vi "Main_007.vi"() -> ()   [LabVIEW 2025]
uses:
  Utility/Universal Utility/TypeDefs_Utility/Cluster_Row-Column.ctl
  9e3f57c0-2ef8-4495-8287-c6a42a5fb955.vi
  Utility/Universal Utility/TypeDefs_Utility/ENUM_4 Directions U-D-L-R.ctl
  Utility/Universal Utility/TypeDefs_Utility/ENUM_8 Directions U-D-L-R.ctl
  <vilib>/gmath/NI_AAL_MathFunc.lvlib
panel:
  out "MATCH":bool
  in  "Select Data":enum32{"Example", "Puzzle"}(tab)
  in  "EX Target":u64=13
  in  "Example Input":u64=6
  in  "Puzzle Input":u64=10001
  in  "Puzzle Target":u64=104743
  out "Answer":u64
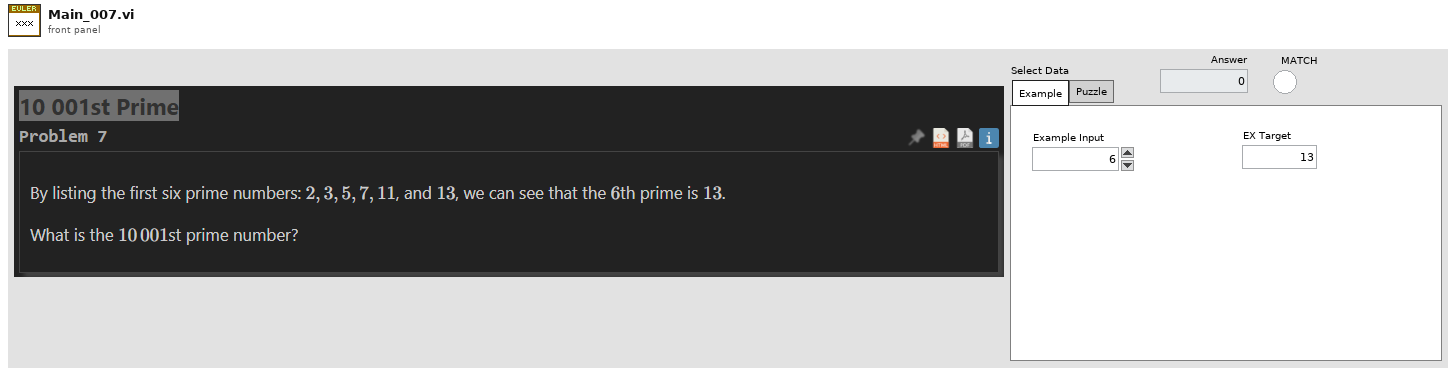
[diagram p1: front panel]
types:
  T1 = typedef "ENUM_8 Directions U-D-L-R.ctl" = enum16{"Up;-1,0", "Up-Right;-1,1", "Right;0,1", "Down-Right;1,1", "Down;1,0", "Down-Left;1,-1", "Left;0,-1", "Up-Left;-1,-1"}
  T2 = typedef "ENUM_4 Directions U-D-L-R.ctl" = enum16{"Up;-1,0", "Right;0,1", "Down;1,0", "Left;0,-1"}
  T3 = typedef "Cluster_Row-Column.ctl" = cluster{"R":i32, "C":i32}
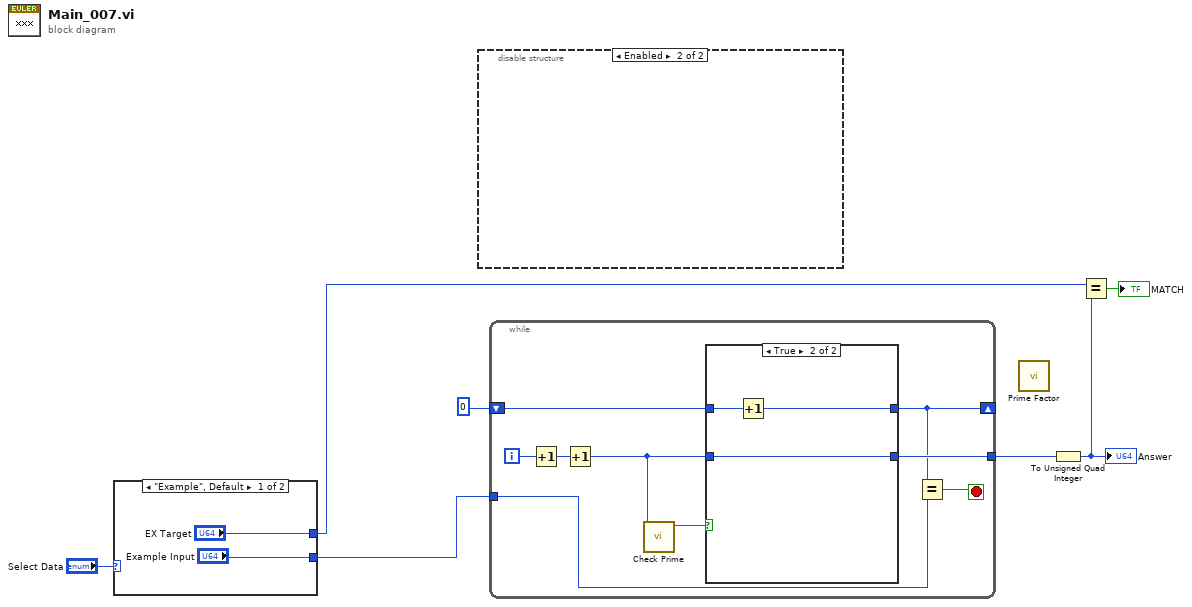
[diagram p0: block diagram]
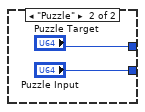
[diagram p3: hidden frame]
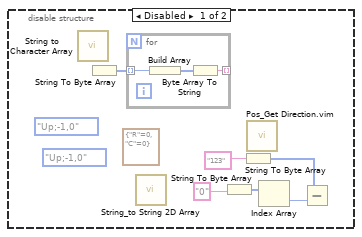
[diagram p4: hidden frame]
diagram:
  n1 = case shown="\"Example\", Default" "Select Data" {
    tunnel: ["Example Input" "Puzzle Input"] -> w3
    tunnel: ["EX Target" "Puzzle Target"] -> w5
    frame "Example", Default {
    }
    frame "Puzzle" {
    }
  }
  n2 = disable-structure shown="Enabled" {
    frame Disabled {
      (unwired) ENUM_8_Directions_U-D-L-R."Up;-1,0" ("Direction 8")
      (unwired) ENUM_4_Directions_U-D-L-R."Up;-1,0" ("Direction")
      (unwired) T3 {"R"=0, "C"=0} ("Position")
      n3 = call "String to Character Array.vi"() -> ()  [unwired: 1 in, 1 out]
      n4 = String To Byte Array() -> (unsigned byte array=w12:u8[])  [unwired: 1 in]
      n5 = for {
        tunnel: w12 -> [w20] mode=indexing
        tunnel: [w18] -> _ mode=indexing
        n6 = Build Array(w20) -> (w19:u8[])
        n7 = Byte Array To String(unsigned byte array=w19) -> (string=w18:string)
      }
      n8 = call "String_to String 2D Array.vi"() -> ()  [unwired: 11 in, 1 out]
      n9 = String To Byte Array(string="0") -> (unsigned byte array=w15:u8[])
      n10 = String To Byte Array(string="123") -> (unsigned byte array=w13:u8[])
      n11 = call "Pos_Get Direction.vim"() -> ()  [unwired: 11 in, 1 out]
      n12 = Index Array(array=w15) -> (element=w14:u8)  [unwired: 1 in]
      n13 = Subtract(x=w13, y=w14) -> ()  [unwired: 1 out]
    }
    frame Enabled {
    }
  }
  n14 = while {
    tunnel: w3 -> [w22]
    shift-right: [w23] -> _
    shift-left: 0 ("x+1") -> [w25]
    tunnel: [w24] -> w1
    i -> [w29]
    stop <- w21 stop-if-true
    n15 = Increment(x=w29) -> (x+1=w28:i32)
    n16 = Increment(x=w28) -> (x+1=w26:i32)
    n17 = call <vilib>:"Check Prime.vi"("n"=w26) -> ("prime?"=w27:bool)  [unwired: 10 in]
    n18 = case shown="True" w27 {
      tunnel: w26 -> [w30 w32]
      tunnel: w25 -> [w31 w34]
      tunnel: [w31 w33] -> w23
      tunnel: [w30 w32] -> w24
      frame False {
      }
      frame True {
        n19 = Increment(x=w34) -> (x+1=w33:i32)
      }
    }
    n20 = Equal?(x=w23, y=w22) -> (x = y?=w21:bool)
  }
  n21 = call <vilib>:"Prime Factor.vi"() -> ()  [unwired: 10 in, 1 out]
  n22 = To Unsigned Quad Integer(1:w1) -> (0:w4:u64)
  "Answer" <- w4
  n23 = Equal?(x=w5, y=w4) -> (x = y?=→"MATCH":bool)
